vi "Choreo_SwerveSample_ModuleForcesY.vi"(11 "ChoreoSwerveSample":T1) -> (3 "ForcesY":dbl[](array[numeric]))   [LabVIEW 2019, in "ChoreoLib.lvlib"]
doc: "Retrieves the Y module forces from a Swerve Trajectory Sample\n\nInputs: \n -- ChoreoSwerveSample - cluster - Swerve sample.\n\nOutputs:\n -- ForcesY - double array - The force on each swerve module in the Y direction in Newtons. Module forces appear in the following order: [FL, FR, BL, BR]."
uses:
  ChoreoLib.lvlib
  TypeDef/ChoreoSwerveSample.ctl
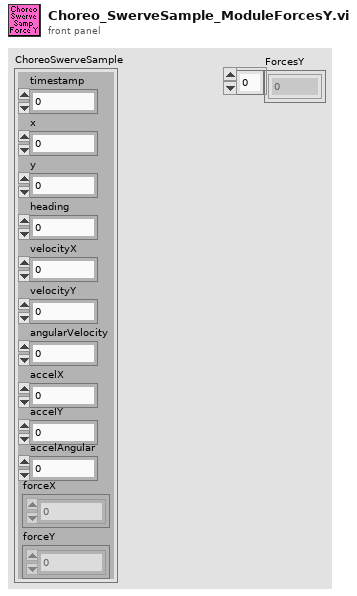
[diagram p1: front panel]
types:
  T1 = typedef "ChoreoLib.lvlib/ChoreoSwerveSample.ctl" = cluster{"timestamp":dbl, "x":dbl, "y":dbl, "heading":dbl, "velocityX":dbl, "velocityY":dbl, "angularVelocity":dbl, "accelX":dbl, "accelY":dbl, "accelAngular":dbl, "forceX":dbl[], "forceY":dbl[]}
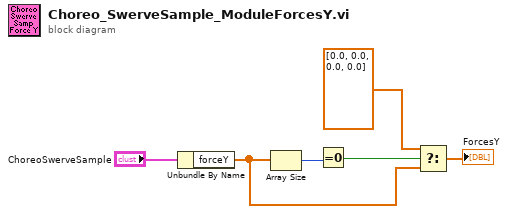
[diagram p0: block diagram]
diagram:
  n1 = Unbundle By Name("ChoreoSwerveSample") -> ("forceY"=w3:dbl[])
  n2 = Array Size(array=w3) -> (size(s)=w5:i32)
  n3 = Equal To 0?(x=w5) -> (x = 0?=w4:bool)
  n4 = Select(t=dbl[] [0.0, 0.0, 0.0, 0.0], s=w4, f=w3) -> (s? t:f=→"ForcesY":dbl[])
